vi "uNotify Update Core.vi"(8 "error in (no error)":errorcluster, 9 "Destination uMsg":refnum<class "uMsg.lvclass">, 10 "uTransport":refnum<class "uTransport.lvclass">, 11 "uNotifyMode in":refnum<class "uNotifyMode.lvclass">) -> (0 "error out":errorcluster)   [LabVIEW 2023, in "uLib.lvlib" / "uNotifyMode.lvclass"]
doc: "Notify the subscriber of an update to the observed event.\n\nThe default parent's behavior is to stream all events in a lossless manner."
uses:
  uNotifyMode.lvclass
  uTransport/uTransport/uTransport.lvclass
  uMsg/uMsg/uMsg.lvclass
  uMsg/uMsg/uMsg.lvclass/uMsg.ctl
  uMsg/uMsg/uMsg Update Timestamp.vi
  uNotifyMode.lvclass/uNotifyMode.ctl
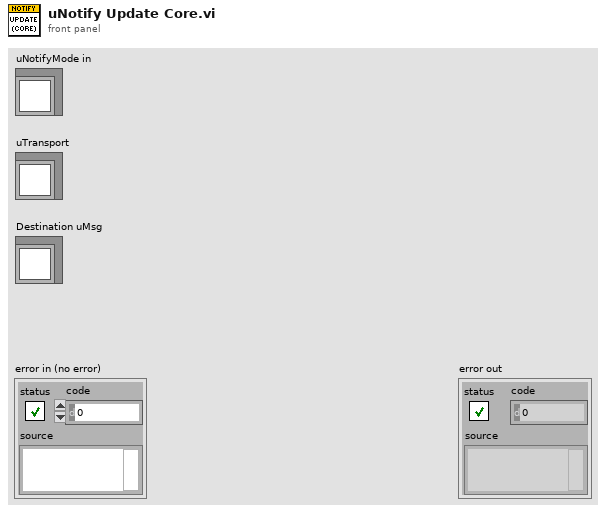
[diagram p1: front panel]
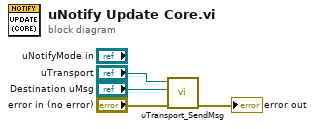
[diagram p0: block diagram]
diagram:
  n1 = call "uTransport_SendMsg.vi"("error in (no error)"="error in (no error)", "Msg"="Destination uMsg", "uTransport in"="uTransport") -> ("error out"=→"error out":errorcluster)  [unwired: 7 in, 1 out]
